vi "init_onemotion.vi"(6 "OneMotion from file":refnum<class "OneMotion.lvclass">, 7 "dimension name":string, 8 "error in (no error)":errorcluster caption="错误输入（无错误）", 9 "CAN node ID":u32, 10 "device index":u32, 11 "OneMotion 输入":refnum<class "OneMotion.lvclass">) -> (0 "error out":errorcluster caption="错误输出", 3 "OneMotion 输出":refnum<class "OneMotion.lvclass">)   [LabVIEW 2016, in "MotionControl_UFO_3DOF.lvlib" / "OneMotion.lvclass"]
uses:
  <userlib>/MotionControl_UFO_3DOF/OneMotion/OneMotion.lvclass
  <userlib>/MotionControl_UFO_3DOF/StepMotor/StepMotor.lvclass
  <userlib>/MotionControl_UFO_3DOF/OneMotion/OneMotion.lvclass/OneMotion.ctl
  <userlib>/MotionControl_UFO_3DOF/LimitSwitch/LimitSwitch.lvclass
  <userlib>/MotionControl_UFO_3DOF/LimitSwitch/LM_ID.ctl
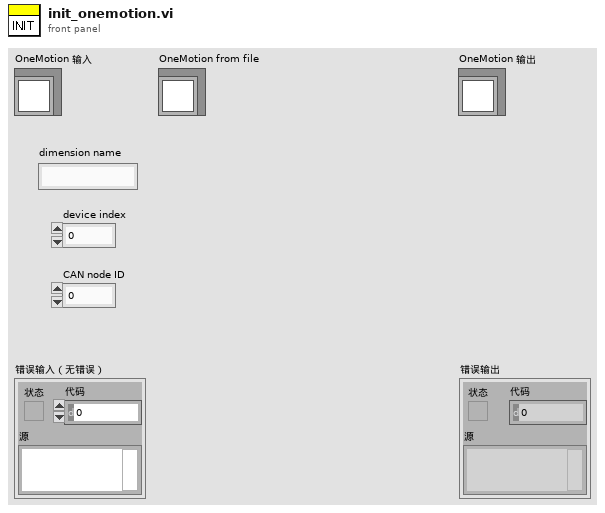
[diagram p1: front panel]
types:
  T1 = typedef "MotionControl_UFO_3DOF.lvlib/LimitSwitch.lvclass/LM_ID.ctl" = i32
  T2 = typedef "MotionControl_UFO_3DOF.lvlib/OneMotion.lvclass/hard limit option.ctl" = enum16{"STOP, and a 0.5s timeout constraint in move", "STOP, and move disabled"}
  T3 = typedef "MotionControl_UFO_3DOF.lvlib/OneMotion.lvclass/unit mode.ctl" = enum16{"motor (pulse)", "linear (mm) or radial (degree)"}
  T4 = typedef "MotionControl_UFO_3DOF.lvlib/OneMotion.lvclass/backlash option.ctl" = enum16{"no backlash compensation", "compensation: from - to +", "compensation: from + to -"}
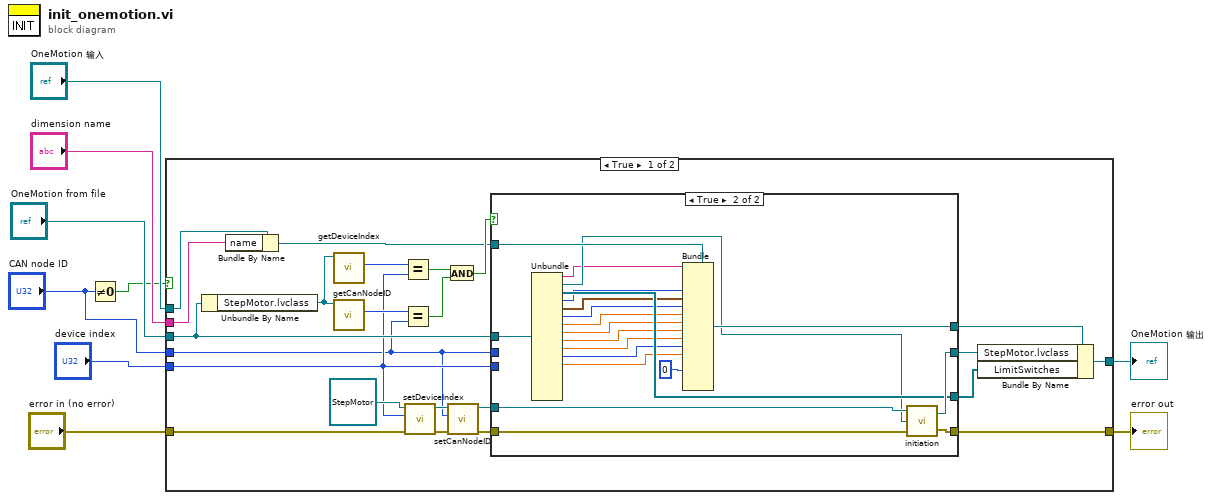
[diagram p0: block diagram]
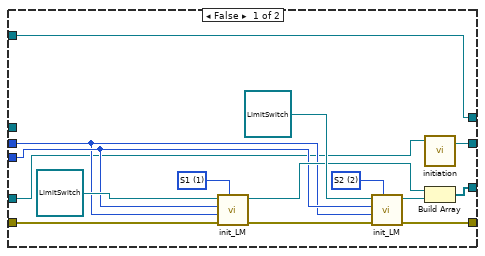
[diagram p2: hidden frame]
diagram:
  n1 = Not Equal To 0?(x="CAN node ID") -> (x != 0?=w1:bool)
  n2 = case shown="True" w1 {
    tunnel: [w26 w68] -> w9
    tunnel: "OneMotion 输入" -> [w32 w69]
    tunnel: [w10 w69] -> w7
    tunnel: "dimension name" -> [w31 _]
    tunnel: "device index" -> [w18 _]
    tunnel: "CAN node ID" -> [w17 _]
    tunnel: "error in (no error)" -> [w28 w68]
    tunnel: "OneMotion from file" -> [w22 _]
    frame True {
      n3 = Unbundle By Name(w22) -> ("StepMotor.lvclass"=w21:refnum<class "StepMotor.lvclass">)
      n4 = Bundle By Name(cluster=w32, "name"=w31) -> (w13:refnum<class "OneMotion.lvclass">)
      n5 = call-dynamic "getDeviceIndex.vi"("StepMotor输入"=w21) -> ("device index"=w20:u32)  [unwired: 8 in, 2 out]
      n6 = call-dynamic "getCanNodeID.vi"("StepMotor输入"=w21) -> ("CAN node ID"=w19:u32)  [unwired: 8 in, 2 out]
      n7 = Equal?(x=w20, y=w18) -> (x = y?=w16:bool)
      n8 = Equal?(x=w19, y=w17) -> (x = y?=w15:bool)
      n9 = call-dynamic "setDeviceIndex.vi"("error in (no error)"=w28, "device index"=w18, "StepMotor输入"=refnum<class "StepMotor.lvclass"> refnum ("StepMotor.lvclass")) -> ("error out"=w27:errorcluster, "StepMotor输出"=w29:refnum<class "StepMotor.lvclass">)  [unwired: 7 in]
      n10 = And(x=w16, y=w15) -> (x .and. y?=w14:bool)
      n11 = call-dynamic "setCanNodeID.vi"("error in (no error)"=w27, "CAN node ID"=w17, "StepMotor输入"=w29) -> ("error out"=w25:errorcluster, "StepMotor输出"=w24:refnum<class "StepMotor.lvclass">)  [unwired: 7 in]
      n12 = case shown="True" w14 {
        tunnel: w22 -> [_ w63]
        tunnel: w18 -> [w40 _]
        tunnel: w17 -> [w39 _]
        tunnel: w25 -> [w38 w65]
        tunnel: [w37 w64] -> w26
        tunnel: [w36 w60] -> w11
        tunnel: w24 -> [w35 w67]
        tunnel: [w34 w66] -> w23
        tunnel: w13 -> [w33 w62]
        tunnel: [w33 w61] -> w12
        frame False {
          w47 = T1 2 items=["none", "S1", "S2", "S3"] ("LM ID")
          w46 = T1 1 items=["none", "S1", "S2", "S3"] ("LM ID")
          n13 = call <userlib>:"init_LM.vi"("LM ID"=w46, "error in (no error)"=w38, "CAN node ID"=w39, "device index"=w40, "LimitSwitch 输入"=refnum<class "LimitSwitch.lvclass"> refnum ("LimitSwitch.lvclass")) -> ("error out"=w44:errorcluster, "LimitSwitch 输出"=w42:refnum<class "LimitSwitch.lvclass">)  [unwired: 5 in]
          n14 = call <userlib>:"init_LM.vi"("LM ID"=w47, "error in (no error)"=w44, "CAN node ID"=w39, "device index"=w40, "LimitSwitch 输入"=refnum<class "LimitSwitch.lvclass"> refnum ("LimitSwitch.lvclass")) -> ("error out"=w37:errorcluster, "LimitSwitch 输出"=w45:refnum<class "LimitSwitch.lvclass">)  [unwired: 5 in]
          n15 = call <userlib>:"initiation.vi"("StepMotor输入"=w35) -> ("StepMotor输出"=w34:refnum<class "StepMotor.lvclass">)  [unwired: 2 in, 1 out]
          n16 = Build Array(w42, w45) -> (w36:refnum<class "LimitSwitch.lvclass">[])
        }
        frame True {
          n17 = Unbundle(w63) -> (w49:string, w59:refnum<class "StepMotor.lvclass">, w60:refnum<class "LimitSwitch.lvclass">[], w58:T2, w57:cluster{"min":dbl, "max":dbl}, w56:T3, w55:dbl, w54:dbl, w53:dbl, w52:dbl, w51:T4, w50:dbl)  [unwired: 4 out]
          n18 = Bundle(cluster=w62, w49, w58, w57, w56, w55, w54, w53, w52, w51, w50, 0) -> (w61:refnum<class "OneMotion.lvclass">)  [unwired: 5 in]
          n19 = call <userlib>:"initiation.vi"("error in (no error)"=w65, "StepMotor from file"=w59, "StepMotor输入"=w67) -> ("error out"=w64:errorcluster, "StepMotor输出"=w66:refnum<class "StepMotor.lvclass">)
        }
      }
      n20 = Bundle By Name(cluster=w12, "StepMotor.lvclass"=w23, "LimitSwitches"=w11) -> (w10:refnum<class "OneMotion.lvclass">)
    }
    frame False {
    }
  }
  "error out" <- w9
  "OneMotion 输出" <- w7
